vi "subHamamatsu_ApplyDAQwaveform.vi"(5 "Camera info":cluster{"Handle in":u32, "Image file path":path}, 6 "Acquisition params":T1={"Sampling rate (Hz)"=0.0, "dt (sec)"=0.0, "total time (sec)"=0.0, "# samples"=0, "Exposure time (ms)"=1000.0, "# frames"=0} {"Exposure time (ms)" format="%0.5f"; "Sampling rate (Hz)" format="%#.3f"}, 7 "Waveform port selection":T2={"Dev2 DO lines"=["Dev2/port0/line3", "Dev2/port0/line5"], "Dev2 AO lines"=["Dev2/ao3", "Dev2/ao5"], "Patch AO line"="Dev1/ao0", "Dev1 AI lines"=["Dev1/ai0", "Dev1/ai8"], "Dev1 timing DO"="Dev1/port0/line1", "Camera timing DI"="Dev1/port0/line0", "Dev1 trigger source"="/Dev1/PFI0", "Dev2 trigger source"="/Dev2/PFI0"}, 8 "Camera in (no error)":errorcluster, 9 "Dev1 AO waveform":waveform(dbl)(graph)={"t0"=timestamp(0 s since 1904-01-01), "dt"=0.1, "Y"=array[20000 elements]}, 10 "Dev2 AO waveform":waveform(dbl)[](graph)=[{"t0"=timestamp(0 s since 1904-01-01), "dt"=0.1, "Y"=array[20000 elements]}, {"t0"=timestamp(0 s since 1904-01-01), "dt"=0.1, "Y"=array[20000 elements]}], 11 "Dev2 DO waveform":digitalwaveform[](graph)=[{"t0"=timestamp(0 s since 1904-01-01), "dt"=0.1, "Y"={"transitions"=[0, 10000, 19999], "data"=[[1], [0], [0]]}}, {"t0"=timestamp(0 s since 1904-01-01), "dt"=0.1, "Y"={"transitions"=[0, 10000, 19999], "data"=[[0], [1], [1]]}}]) -> (0 "Camera out":errorcluster, 2 "AI Waveform":dbl[][](graph), 3 "Camera timging DI":digitalwaveform(graph))   [LabVIEW 2015]
uses:
  <vilib>/DAQmx/write.llb/DAQmx Write (Analog Wfm 1Chan NSamp).vi
  <vilib>/DAQmx/write.llb/DAQmx Write (Analog 1D Wfm NChan NSamp).vi
  <vilib>/DAQmx/write.llb/DAQmx Write (Digital 1D Wfm NChan NSamp).vi
  <vilib>/DAQmx/write.llb/DAQmx Write (Digital Wfm 1Chan NSamp).vi
  <vilib>/DAQmx/read.llb/DAQmx Read (Analog 2D DBL NChan NSamp).vi
  <vilib>/DAQmx/read.llb/DAQmx Read (Digital Wfm 1Chan NSamp).vi
  <vilib>/DAQmx/create/channels.llb/DAQmx Create Channel (DO-Digital Output).vi
  <vilib>/Waveform/DWDTOps.llb/DWDT Analog to Digital.vi
  <vilib>/DAQmx/create/channels.llb/DAQmx Create Channel (DI-Digital Input).vi
  <vilib>/DAQmx/configure/timing.llb/DAQmx Timing (Sample Clock).vi
  <vilib>/DAQmx/create/channels.llb/DAQmx Create Channel (AO-Voltage-Basic).vi
  <vilib>/DAQmx/miscellaneous.llb/DAQmx Fill In Error Info.vi
  <vilib>/DAQmx/create/channels.llb/DAQmx Create Channel (AI-Voltage-Basic).vi
  <vilib>/DAQmx/configure/trigger.llb/DAQmx Start Trigger (Digital Edge).vi
  <vilib>/Waveform/DWDTOps.llb/DWDT Uncompress Digital.vi
  <vilib>/DAQmx/configure/trigger.llb/DAQmx Start Trigger (None).vi
  <resource>/objmgr/daqmx.rc
panel:
  out "Dev1 SampClk.Rate":dbl format="%#.3f"
  out "Dev2 SampClk.Rate":dbl format="%#.3f"
  out "Dev1 timing DO":digitalwaveform(graph)={"t0"=timestamp(0 s since 1904-01-01), "dt"=0.1, "Y"={"transitions"=[0, 19999], "data"=[[1], [1]]}}
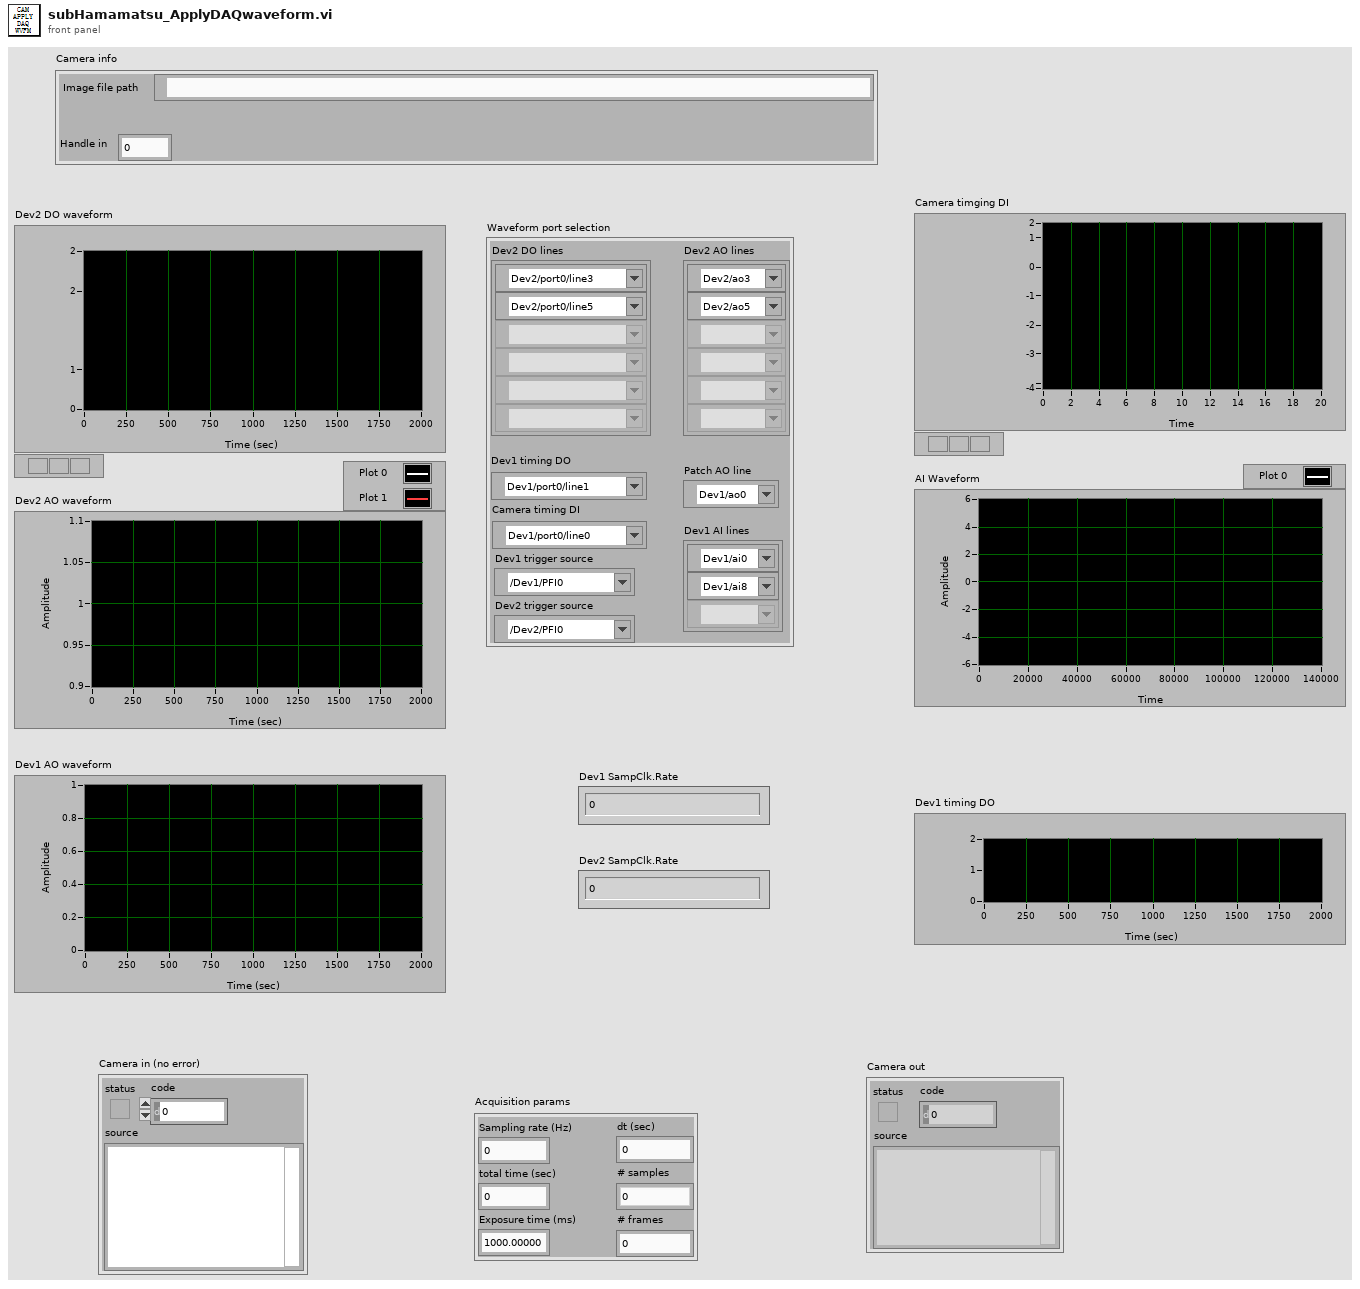
[diagram p1: front panel]
types:
  T1 = cluster{"Sampling rate (Hz)":dbl, "dt (sec)":dbl, "total time (sec)":dbl, "# samples":i32, "Exposure time (ms)":dbl, "# frames":i32}
  T2 = cluster{"Dev2 DO lines":tag[], "Dev2 AO lines":tag[], "Patch AO line":tag, "Dev1 AI lines":tag[], "Dev1 timing DO":tag, "Camera timing DI":tag, "Dev1 trigger source":tag, "Dev2 trigger source":tag}
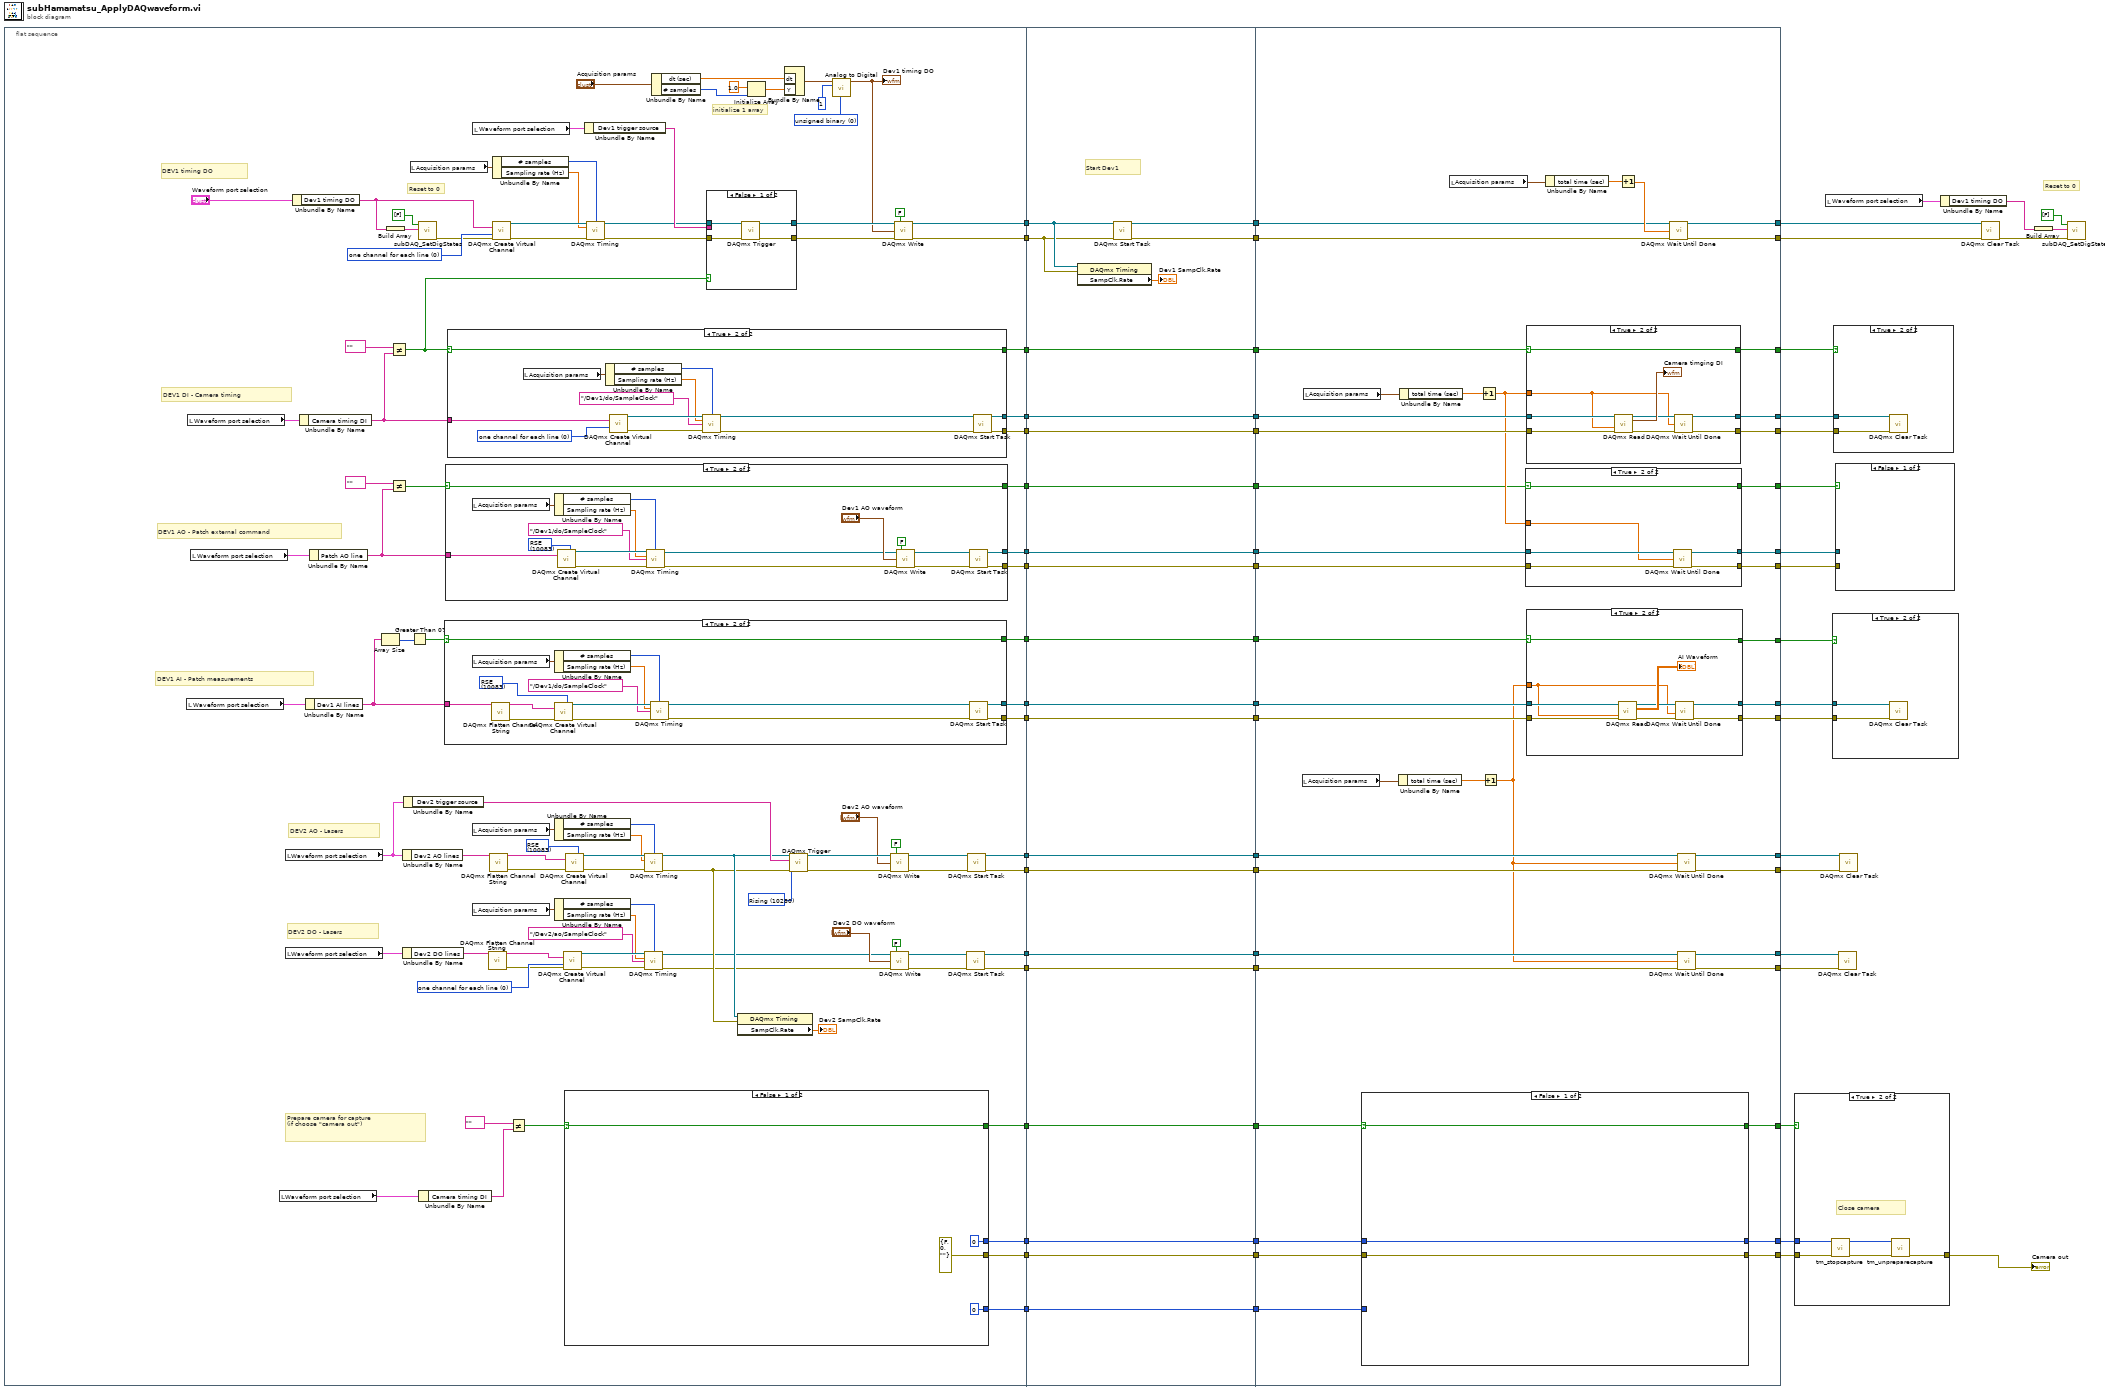
[diagram p0: block diagram]
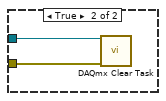
[diagram p5: hidden frame]
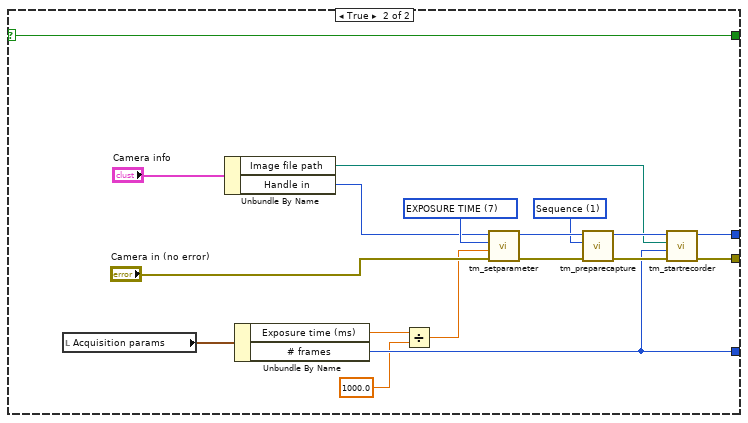
[diagram p6: hidden frame]
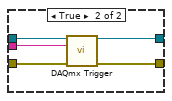
[diagram p7: hidden frame]
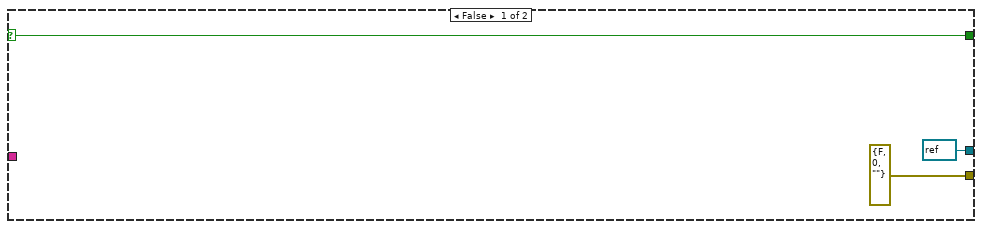
[diagram p8: hidden frame]
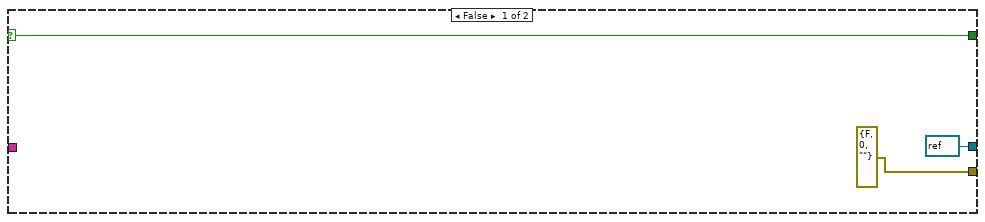
[diagram p9: hidden frame]
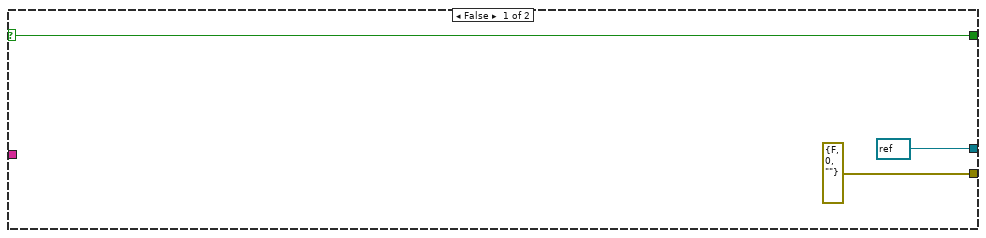
[diagram p10: hidden frame]
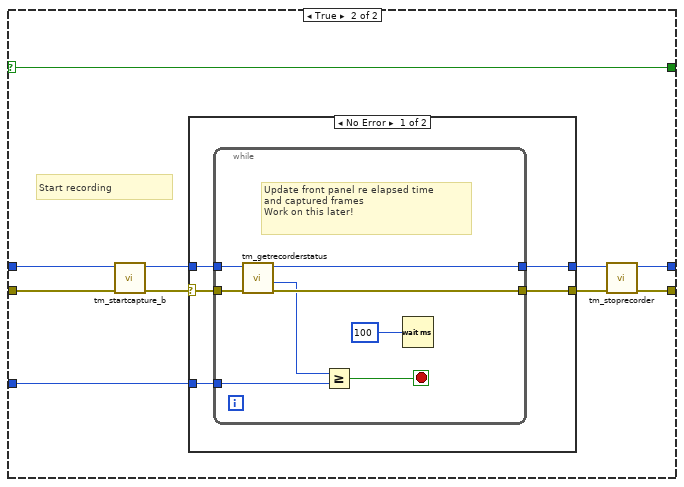
[diagram p11: hidden frame]
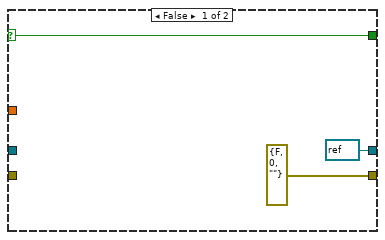
[diagram p13: hidden frame]
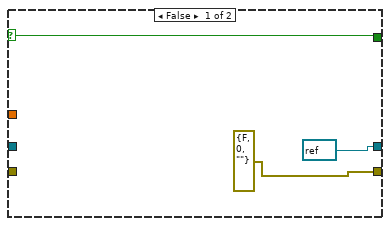
[diagram p14: hidden frame]
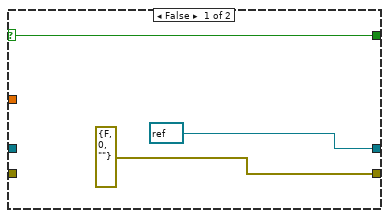
[diagram p15: hidden frame]
diagram:
  # "Reset to 0"
  n1 = flat-sequence {
    tunnel: [w148] -> w39
    tunnel: [w69] -> w37
    tunnel: [w68] -> w35
    tunnel: [w131] -> w34
    tunnel: [w129] -> w32
    tunnel: [w128] -> w30
    tunnel: [w126] -> w28
    tunnel: [w125] -> w26
    tunnel: [w122] -> w24
    tunnel: [w121] -> w22
    tunnel: [w118] -> w20
    tunnel: [w117] -> w18
    tunnel: [w112] -> w16
    tunnel: [w111] -> w14
    tunnel: [w98] -> w12
    tunnel: [w79] -> w10
    tunnel: [w75] -> w8
    tunnel: [w72] -> w6
    tunnel: [w63] -> w2
    tunnel: w39 -> [w269]
    tunnel: [w269] -> w38
    tunnel: w37 -> [w250]
    tunnel: [w252] -> w36
    tunnel: w35 -> [w249]
    tunnel: w34 -> [w268]
    tunnel: [w268] -> w33
    tunnel: w32 -> [w267]
    tunnel: [w267] -> w31
    tunnel: w30 -> [w266]
    tunnel: [w266] -> w29
    tunnel: w28 -> [w265]
    tunnel: [w265] -> w27
    tunnel: w26 -> [w264]
    tunnel: [w264] -> w25
    tunnel: w24 -> [w263]
    tunnel: [w263] -> w23
    tunnel: w22 -> [w262]
    tunnel: [w262] -> w21
    tunnel: w20 -> [w261]
    tunnel: [w261] -> w19
    tunnel: w18 -> [w260]
    tunnel: [w260] -> w17
    tunnel: w16 -> [w259]
    tunnel: [w259] -> w15
    tunnel: w14 -> [w258]
    tunnel: [w258] -> w13
    tunnel: w12 -> [w257]
    tunnel: [w257] -> w11
    tunnel: w10 -> [w256]
    tunnel: [w256] -> w9
    tunnel: w8 -> [w255]
    tunnel: [w255] -> w7
    tunnel: w6 -> [w254]
    tunnel: [w254] -> w5
    tunnel: [w251] -> w4
    tunnel: [w248] -> w3
    tunnel: w2 -> [w248]
    tunnel: w38 -> [w311]
    tunnel: w36 -> [w273]
    tunnel: w33 -> [w310]
    tunnel: w31 -> [w309]
    tunnel: w29 -> [w308]
    tunnel: w27 -> [w306]
    tunnel: w25 -> [w307]
    tunnel: w23 -> [w305]
    tunnel: w21 -> [w304]
    tunnel: w19 -> [w303]
    tunnel: w17 -> [w302]
    tunnel: w15 -> [w315]
    tunnel: w13 -> [w314]
    tunnel: [w313] -> w56
    tunnel: [w312] -> w55
    tunnel: [w301] -> w54
    tunnel: [w300] -> w53
    tunnel: [w299] -> w52
    tunnel: [w298] -> w51
    tunnel: [w297] -> w50
    tunnel: [w296] -> w49
    tunnel: [w295] -> w48
    tunnel: [w294] -> w47
    tunnel: [w293] -> w46
    tunnel: [w292] -> w45
    tunnel: [w291] -> w44
    tunnel: [w290] -> w43
    tunnel: w11 -> [w289]
    tunnel: w9 -> [w279]
    tunnel: [w278] -> w42
    tunnel: w7 -> [w277]
    tunnel: [w276] -> w41
    tunnel: w5 -> [w275]
    tunnel: [w274] -> w40
    tunnel: w4 -> [w272]
    tunnel: w3 -> [w271]
    tunnel: [w270] -> w1
    frame #0 {
      w94 = 10083 items=["Default"=-1, "RSE"=10083, "Differential"=10106, "Pseudodifferential"=12529] ("output terminal configuration")
      w97 = 10280 items=["Rising"=10280, "Falling"=10171] ("edge")
      w110 = u16 0 items=["unsigned binary", "offset binary", "2's complement"] ("data format (offset binary)")
      w140 = 0 items=["one channel for each line", "one channel for all lines"] ("line grouping")
      w162 = 0 items=["one channel for each line", "one channel for all lines"] ("line grouping")
      # "Prepare camera for capture\n(if choose \"camera out\")"
      # "Reset to 0"
      # "DEV2 DO - Lasers"
      # "DEV2 AO - Lasers"
      # "DEV1 AI - Patch measurements"
      # "DEV1 AO - Patch external command"
      # "DEV1 DI - Camera timing"
      # "DEV1 timing DO"
      # "initialize 1 array"
      n2 = local read "Waveform port selection"() -> (w127:T2)
      n3 = local read "Waveform port selection"() -> (w132:T2)
      n4 = local read "Waveform port selection"() -> (w83:T2)
      n5 = local read "Waveform port selection"() -> (w65:T2)
      n6 = local read "Waveform port selection"() -> (w109:T2)
      n7 = local read "Waveform port selection"() -> (w120:T2)
      n8 = Unbundle By Name("Waveform port selection") -> ("Dev1 timing DO"=w115:tag)
      n9 = Unbundle By Name(w132) -> ("Camera timing DI"=w73:tag)
      n10 = Unbundle By Name(w127) -> ("Dev1 AI lines"=w78:tag[])
      n11 = Unbundle By Name(w83) -> ("Patch AO line"=w82:tag)
      n12 = Array Size(array=w78) -> (size(s)=w77:i32)
      n13 = Build Array(w115) -> (w114:tag[])
      n14 = Not Equal?(x=tag "" ("Patch amplifier"), y=w73) -> (x != y?=w70:bool)
      n15 = Not Equal?(x=tag "" ("Patch amplifier"), y=w82) -> (x != y?=w80:bool)
      n16 = Unbundle By Name(w109) -> ("Dev2 AO lines"=w123:tag[])
      n17 = Unbundle By Name(w120) -> ("Dev2 DO lines"=w119:tag[])
      n18 = Unbundle By Name(w109) -> ("Dev2 trigger source"=w108:tag)
      n19 = local read "Acquisition params"() -> (w86:T1)
      n20 = Greater Than 0?(x=w77) -> (x > 0?=w76:bool)
      n21 = call "subDAQ_SetDigStates.vi"("Digital line array"=w114, "Digital States (Value) array"=bool[] [FALSE] ("Digital state array")) -> ("Error out"=w116:errorcluster)  [unwired: 9 in]
      n22 = Unbundle By Name(w65) -> ("Camera timing DI"=w67:tag)
      n23 = case shown="True" w76 {
        selector: w76 -> [w212 w213]
        tunnel: w78 -> [_ w223]
        tunnel: [errorcluster {"status"=FALSE, "code"=0, "source"=""} ("error out") w222] -> w126
        tunnel: [refnum<k21> refnum ("task out") w221] -> w125
        tunnel: [w212 w213] -> w75
        frame False {
        }
        frame True {
          w216 = 10083 items=["Default"=-1, "RSE"=10083, "NRSE"=10078, "Differential"=10106, "Pseudodifferential"=12529] ("input terminal configuration")
          n24 = local read "Acquisition params"() -> (w219:T1)
          n25 = call <vilib>:"DAQmx Flatten Channel String.vi"("names in"=w223) -> ("names out"=w227:string, "error out"=w226:errorcluster)  [unwired: 13 in]
          n26 = Unbundle By Name(w219) -> ("# samples"=w217:i32, "Sampling rate (Hz)"=w218:dbl)
          n27 = call-poly <vilib>:"DAQmx Create Virtual Channel.vi"("input terminal configuration"=w216, "physical channels"=w227, "error in"=w226) -> ("task out"=w224:refnum<k21>, "error out"=w225:errorcluster)  [unwired: 11 in]
          n28 = call-poly <vilib>:"DAQmx Timing.vi"("task/channels in"=w224, "samples per channel"=w217, "rate"=w218, "source"=tag "/Dev1/do/SampleClock", "error in"=w225) -> ("task out"=w215:refnum<k21>, "error out"=w214:errorcluster)  [unwired: 9 in]
          n29 = call <vilib>:"DAQmx Start Task.vi"("task/channels in"=w215, "error in"=w214) -> ("task out"=w221:refnum<k21>, "error out"=w222:errorcluster)  [unwired: 12 in]
        }
      }
      n30 = case shown="True" w80 {
        selector: w80 -> [w230 w231]
        tunnel: [refnum<k21> refnum ("task out") w241] -> w129
        tunnel: [errorcluster {"status"=FALSE, "code"=0, "source"=""} ("error out") w240] -> w128
        tunnel: w82 -> [_ w232]
        tunnel: [w230 w231] -> w79
        frame False {
        }
        frame True {
          w235 = 10083 items=["Default"=-1, "RSE"=10083, "Differential"=10106, "Pseudodifferential"=12529] ("output terminal configuration")
          n31 = local read "Acquisition params"() -> (w236:T1)
          n32 = Unbundle By Name(w236) -> ("# samples"=w238:i32, "Sampling rate (Hz)"=w237:dbl)
          n33 = call-poly <vilib>:"DAQmx Create Virtual Channel.vi"("output terminal configuration"=w235, "physical channels"=w232) -> ("task out"=w244:refnum<k21>, "error out"=w246:errorcluster)  [unwired: 12 in]
          n34 = call-poly <vilib>:"DAQmx Timing.vi"("task/channels in"=w244, "samples per channel"=w238, "rate"=w237, "source"=tag "/Dev1/do/SampleClock", "error in"=w246) -> ("task out"=w234:refnum<k21>, "error out"=w233:errorcluster)  [unwired: 9 in]
          n35 = call-poly <vilib>:"DAQmx Write.vi"("task/channels in"=w234, "auto start"=FALSE, "data"="Dev1 AO waveform", "error in"=w233) -> ("task out"=w245:refnum<k21>, "error out"=w242:errorcluster)  [unwired: 9 in, 1 out]
          n36 = call <vilib>:"DAQmx Start Task.vi"("task/channels in"=w245, "error in"=w242) -> ("task out"=w241:refnum<k21>, "error out"=w240:errorcluster)  [unwired: 12 in]
        }
      }
      n37 = case shown="True" w70 {
        selector: w70 -> [w196 w197]
        tunnel: [refnum<k21> refnum ("task out") w206] -> w148
        tunnel: w73 -> [_ w205]
        tunnel: [errorcluster {"status"=FALSE, "code"=0, "source"=""} ("error out") w204] -> w131
        tunnel: [w196 w197] -> w72
        frame False {
        }
        frame True {
          w209 = 0 items=["one channel for each line", "one channel for all lines"] ("line grouping")
          n38 = local read "Acquisition params"() -> (w202:T1)
          n39 = Unbundle By Name(w202) -> ("# samples"=w201:i32, "Sampling rate (Hz)"=w200:dbl)
          n40 = call-poly <vilib>:"DAQmx Create Virtual Channel.vi"("lines"=w205, "line grouping"=w209) -> ("task out"=w208:refnum<k21>, "error out"=w207:errorcluster)  [unwired: 12 in]
          n41 = call-poly <vilib>:"DAQmx Timing.vi"("task/channels in"=w208, "samples per channel"=w201, "rate"=w200, "source"=tag "/Dev1/do/SampleClock", "error in"=w207) -> ("task out"=w199:refnum<k21>, "error out"=w198:errorcluster)  [unwired: 9 in]
          n42 = call <vilib>:"DAQmx Start Task.vi"("task/channels in"=w199, "error in"=w198) -> ("task out"=w206:refnum<k21>, "error out"=w204:errorcluster)  [unwired: 12 in]
        }
      }
      n43 = local read "Acquisition params"() -> (w104:T1)
      n44 = local read "Acquisition params"() -> (w103:T1)
      n45 = local read "Waveform port selection"() -> (w71:T2)
      n46 = call <vilib>:"DAQmx Flatten Channel String.vi"("names in"=w119) -> ("names out"=w160:string, "error out"=w159:errorcluster)  [unwired: 13 in]
      n47 = call <vilib>:"DAQmx Flatten Channel String.vi"("names in"=w123) -> ("names out"=w144:string, "error out"=w145:errorcluster)  [unwired: 13 in]
      n48 = Unbundle By Name(w86) -> ("# samples"=w85:i32, "Sampling rate (Hz)"=w84:dbl)
      n49 = call-poly <vilib>:"DAQmx Create Virtual Channel.vi"("lines"=w115, "line grouping"=w140, "error in"=w116) -> ("task out"=w141:refnum<k21>, "error out"=w143:errorcluster)  [unwired: 11 in]
      n50 = Not Equal?(x=tag "" ("Patch amplifier"), y=w67) -> (x != y?=w64:bool)
      n51 = Unbundle By Name(w104) -> ("# samples"=w99:i32, "Sampling rate (Hz)"=w100:dbl)
      n52 = Unbundle By Name(w103) -> ("# samples"=w102:i32, "Sampling rate (Hz)"=w101:dbl)
      n53 = call-poly <vilib>:"DAQmx Create Virtual Channel.vi"("lines"=w160, "line grouping"=w162, "error in"=w159) -> ("task out"=w161:refnum<k21>, "error out"=w156:errorcluster)  [unwired: 11 in]
      n54 = case shown="False" w64 {
        selector: w64 -> [w163 w167]
        tunnel: [u32 0 ("Handle out") w177] -> w112
        tunnel: [errorcluster {"status"=FALSE, "code"=0, "source"=""} ("error out") w176] -> w111
        tunnel: [0 ("# frames") w172] -> w98
        tunnel: [w163 w167] -> w63
        frame False {
        }
        frame True {
          w181 = 7 items=["BINNING"=1, "BITS PER CHANNEL"=2, "ACTIVE VIEW INDEX"=3, "CCD MODE"=4, "SENSOR MODE"=5, "READOUT MODE"=6, "EXPOSURE TIME"=7, "CONTRAST GAIN"=8, "CONTRAST OFFSET"=9, "LIGHT MODE"=10, "SENSITIVITY"=11, "WHITE BALANCE"=12, "PHOTON IMAGING MODE"=13, "HIGH DYNAMIC RANGE MODE"=14, "TRIGGER SOURCE"=15, "TRIGGER ACTIVE"=16, "TRIGGER MODE"=17, "TRIGGER POLARITY"=18, "TRIGGER GLOBAL EXPOSURE"=19, "FIRST TRIGGER BEHAVIOR"=20, "TRIGGER TIMES"=21, "OUTPUT TRIGGER POLARITY"=22, "OUTPUT TRIGGER DELAY"=23, "OUTPUT TRIGGER PERIOD"=24, "TEMPERATURE"=25, "TEMPERATURE TARGET"=26, "SENSOR COOLER FAN"=27, "MECHANICAL SHUTTER"=28, "BACK FOCUS POSITION"=29, "FRAMEBUNDLE MODE"=30, "FRAMEBUNDLE NUMBER"=31, "LINEBUNDLE HEIGHT"=32, "TRIGGER CONNECTOR"=33, "IMAGE PIXEL TYPE"=34] ("Parameter")
          w178 = 1 items=["Snap", "Sequence"] ("Capture mode")
          n55 = local read "Acquisition params"() -> (w173:T1)
          n56 = Unbundle By Name("Camera info") -> ("Image file path"=w174:path, "Handle in"=w171:u32)
          n57 = Unbundle By Name(w173) -> ("Exposure time (ms)"=w169:dbl, "# frames"=w172:i32)
          n58 = Divide(x=w169, y=1000.0) -> (x/y=w170:dbl)
          n59 = call "tm_setparameter.vi"("error in (no error)"="Camera in (no error)", "Value in"=w170, "Parameter"=w181, "Handle in"=w171) -> ("error out"=w183:errorcluster, "Handle out"=w182:u32)  [unwired: 6 in]
          n60 = call "tm_preparecapture.vi"("error in (no error)"=w183, "Capture mode"=w178, "Handle in"=w182) -> ("error out"=w179:errorcluster, "Handle out"=w180:u32)  [unwired: 5 in, 2 out]
          n61 = call "tm_startrecorder.vi"("error in (no error)"=w179, "frames"=w172, "File"=w174, "Handle in"=w180) -> ("error out"=w176:errorcluster, "Handle out"=w177:u32)  [unwired: 6 in]
        }
      }
      n62 = call-poly <vilib>:"DAQmx Create Virtual Channel.vi"("output terminal configuration"=w94, "physical channels"=w144, "error in"=w145) -> ("task out"=w155:refnum<k21>, "error out"=w151:errorcluster)  [unwired: 11 in]
      n63 = Unbundle By Name(w71) -> ("Dev1 trigger source"=w106:tag)
      n64 = call-poly <vilib>:"DAQmx Timing.vi"("task/channels in"=w141, "samples per channel"=w85, "rate"=w84, "error in"=w143) -> ("task out"=w90:refnum<k21>, "error out"=w89:errorcluster)  [unwired: 10 in]
      n65 = call-poly <vilib>:"DAQmx Timing.vi"("task/channels in"=w161, "samples per channel"=w102, "rate"=w101, "source"=tag "/Dev2/ao/SampleClock", "error in"=w156) -> ("task out"=w88:refnum<k21>, "error out"=w87:errorcluster)  [unwired: 9 in]
      n66 = call-poly <vilib>:"DAQmx Timing.vi"("task/channels in"=w155, "samples per channel"=w99, "rate"=w100, "error in"=w151) -> ("task out"=w92:refnum<k21>, "error out"=w91:errorcluster)  [unwired: 10 in]
      n67 = Unbundle By Name("Acquisition params") -> ("dt (sec)"=w95:dbl, "# samples"=w96:i32)
      n68 = case shown="False" w70 {
        tunnel: [w186 w193] -> w139
        tunnel: [w187 w192] -> w138
        tunnel: w106 -> [_ w191]
        tunnel: w90 -> [w188 w190]
        tunnel: w89 -> [w185 w189]
        frame False {
          n69 = call-poly <vilib>:"DAQmx Trigger.vi"("task/channels in"=w188, "error in"=w185) -> ("task out"=w187:refnum<k21>, "error out"=w186:errorcluster)  [unwired: 12 in]
        }
        frame True {
          n70 = call-poly <vilib>:"DAQmx Trigger.vi"("task/channels in"=w190, "source"=w191, "error in"=w189) -> ("task out"=w192:refnum<k21>, "error out"=w193:errorcluster)  [unwired: 11 in]
        }
      }
      n71 = property class="DAQmx Timing"(reference=w92, error in=w91) -> ("SampClk.Rate"=→"Dev2 SampClk.Rate":dbl)  [unwired: 2 out]
      n72 = Initialize Array(1.0 ("element"), w96) -> (w136:dbl[])
      n73 = Bundle By Name("dt"=w95, "Y"=w136) -> (w134:waveform(dbl))  [unwired: 1 in]
      n74 = call-poly <vilib>:"DAQmx Trigger.vi"("task/channels in"=w92, "source"=w108, "edge"=w97, "error in"=w91) -> ("task out"=w153:refnum<k21>, "error out"=w152:errorcluster)  [unwired: 10 in]
      n75 = call-poly <vilib>:"Analog to Digital.vi"("data format (offset binary)"=w110, "resolution (16 bit)"=1, "analog waveform"=w134) -> ("digital waveform"=w133:digitalwaveform)  [unwired: 5 in, 3 out]
      "Dev1 timing DO" <- w133
      n76 = call-poly <vilib>:"DAQmx Write.vi"("task/channels in"=w153, "auto start"=FALSE, "data"="Dev2 AO waveform", "error in"=w152) -> ("task out"=w154:refnum<k21>, "error out"=w124:errorcluster)  [unwired: 9 in, 1 out]
      n77 = call-poly <vilib>:"DAQmx Write.vi"("task/channels in"=w88, "auto start"=FALSE, "data"="Dev2 DO waveform", "error in"=w87) -> ("task out"=w158:refnum<k21>, "error out"=w130:errorcluster)  [unwired: 9 in, 1 out]
      n78 = call-poly <vilib>:"DAQmx Write.vi"("task/channels in"=w138, "auto start"=FALSE, "data"=w133, "error in"=w139) -> ("task out"=w69:refnum<k21>, "error out"=w68:errorcluster)  [unwired: 9 in, 1 out]
      n79 = call <vilib>:"DAQmx Start Task.vi"("task/channels in"=w158, "error in"=w130) -> ("task out"=w118:refnum<k21>, "error out"=w117:errorcluster)  [unwired: 12 in]
      n80 = call <vilib>:"DAQmx Start Task.vi"("task/channels in"=w154, "error in"=w124) -> ("task out"=w122:refnum<k21>, "error out"=w121:errorcluster)  [unwired: 12 in]
    }
    frame #1 {
      # "Start Dev1"
      n81 = property class="DAQmx Timing"(reference=w250, error in=w249) -> ("SampClk.Rate"=→"Dev1 SampClk.Rate":dbl)  [unwired: 2 out]
      n82 = call <vilib>:"DAQmx Start Task.vi"("task/channels in"=w250, "error in"=w249) -> ("task out"=w252:refnum<k21>, "error out"=w251:errorcluster)  [unwired: 12 in]
    }
    frame #2 {
      n83 = local read "Acquisition params"() -> (w281:T1)
      n84 = local read "Acquisition params"() -> (w283:T1)
      n85 = case shown="False" w271 {
        selector: w271 -> [w318 w319]
        tunnel: w315 -> [w317 w324]
        tunnel: w314 -> [w316 w323]
        tunnel: [w317 w322] -> w313
        tunnel: [w316 w321] -> w312
        tunnel: w289 -> [_ w320]
        tunnel: [w318 w319] -> w270
        frame False {
        }
        frame True {
          # "Start recording"
          n86 = call "tm_startcapture_b.vi"("error in (no error)"=w323, "Handle in"=w324) -> ("error out"=w325:errorcluster, "Handle out"=w326:u32)  [unwired: 8 in]
          n87 = case shown="No Error" w325 {
            selector: w325 -> [w333 w342]
            tunnel: w326 -> [w332 w343]
            tunnel: [w330 w343] -> w328
            tunnel: [w331 w342] -> w327
            tunnel: w320 -> [w329 _]
            frame No Error {
              n88 = while {
                tunnel: w333 -> [w340]
                tunnel: w332 -> [w339]
                tunnel: [w338] -> w331
                tunnel: [w341] -> w330
                tunnel: w329 -> [w334]
                stop <- w337 stop-if-true
                # "Update front panel re elapsed time\nand captured frames\nWork on this later!"
                n89 = call "tm_getrecorderstatus.vi"("error in (no error)"=w340, "Handle"=w339) -> ("error out"=w338:errorcluster, "Count"=w335:i32, "Handle"=w341:u32)  [unwired: 6 in, 1 out]
                n90 = Greater Or Equal?(x=w335, y=w334) -> (x >= y?=w337:bool)
                n91 = Wait (ms)(milliseconds to wait=u32 100) -> ()  [unwired: 1 out]
              }
            }
            frame Error {
            }
          }
          n92 = call "tm_stoprecorder.vi"("error in (no error)"=w327, "Handle in"=w328) -> ("error out"=w321:errorcluster, "Handle out"=w322:u32)  [unwired: 8 in]
        }
      }
      n93 = Unbundle By Name(w281) -> ("total time (sec)"=w280:dbl)
      n94 = Unbundle By Name(w283) -> ("total time (sec)"=w282:dbl)
      n95 = local read "Acquisition params"() -> (w285:T1)
      n96 = Increment(x=w282) -> (x+1=w287:dbl)
      n97 = Increment(x=w280) -> (x+1=w286:dbl)
      n98 = case shown="True" w279 {
        selector: w279 -> [w370 w372]
        tunnel: w309 -> [_ w376]
        tunnel: w308 -> [_ w375]
        tunnel: [refnum<k21> refnum ("task out") w374] -> w297
        tunnel: [errorcluster {"status"=FALSE, "code"=0, "source"=""} ("error out") w373] -> w296
        tunnel: w287 -> [_ w371]
        tunnel: [w370 w372] -> w278
        frame False {
        }
        frame True {
          n99 = call <vilib>:"DAQmx Wait Until Done.vi"("task/channels in"=w376, "timeout (sec)"=w371, "error in"=w375) -> ("task out"=w374:refnum<k21>, "error out"=w373:errorcluster)  [unwired: 11 in]
        }
      }
      n100 = case shown="True" w275 {
        selector: w275 -> [w346 w347]
        tunnel: w311 -> [_ w352]
        tunnel: w310 -> [_ w351]
        tunnel: [refnum<k21> refnum ("task out") w350] -> w299
        tunnel: [errorcluster {"status"=FALSE, "code"=0, "source"=""} ("error out") w349] -> w298
        tunnel: w287 -> [_ w348]
        tunnel: [w346 w347] -> w274
        frame False {
        }
        frame True {
          n101 = call-poly <vilib>:"DAQmx Read.vi"("task/channels in"=w352, "timeout"=w348, "error in"=w351) -> ("task out"=w353:refnum<k21>, "data"=→"Camera timging DI":digitalwaveform, "error out"=w355:errorcluster)  [unwired: 10 in]
          n102 = call <vilib>:"DAQmx Wait Until Done.vi"("task/channels in"=w353, "timeout (sec)"=w348, "error in"=w355) -> ("task out"=w350:refnum<k21>, "error out"=w349:errorcluster)  [unwired: 11 in]
        }
      }
      n103 = case shown="True" w277 {
        selector: w277 -> [w358 w360]
        tunnel: w307 -> [_ w364]
        tunnel: w306 -> [_ w363]
        tunnel: [refnum<k21> refnum ("task out") w362] -> w295
        tunnel: [errorcluster {"status"=FALSE, "code"=0, "source"=""} ("error out") w361] -> w294
        tunnel: w286 -> [_ w359]
        tunnel: [w358 w360] -> w276
        frame False {
        }
        frame True {
          n104 = call-poly <vilib>:"DAQmx Read.vi"("task/channels in"=w364, "timeout"=w359, "error in"=w363) -> ("task out"=w365:refnum<k21>, "data"=→"AI Waveform":dbl[][], "error out"=w366:errorcluster)  [unwired: 10 in]
          n105 = call <vilib>:"DAQmx Wait Until Done.vi"("task/channels in"=w365, "timeout (sec)"=w359, "error in"=w366) -> ("task out"=w362:refnum<k21>, "error out"=w361:errorcluster)  [unwired: 11 in]
        }
      }
      n106 = Unbundle By Name(w285) -> ("total time (sec)"=w284:dbl)
      n107 = Increment(x=w284) -> (x+1=w288:dbl)
      n108 = call <vilib>:"DAQmx Wait Until Done.vi"("task/channels in"=w273, "timeout (sec)"=w288, "error in"=w272) -> ("task out"=w301:refnum<k21>, "error out"=w300:errorcluster)  [unwired: 11 in]
      n109 = call <vilib>:"DAQmx Wait Until Done.vi"("task/channels in"=w305, "timeout (sec)"=w286, "error in"=w304) -> ("task out"=w293:refnum<k21>, "error out"=w292:errorcluster)  [unwired: 11 in]
      n110 = call <vilib>:"DAQmx Wait Until Done.vi"("task/channels in"=w303, "timeout (sec)"=w286, "error in"=w302) -> ("task out"=w291:refnum<k21>, "error out"=w290:errorcluster)  [unwired: 11 in]
    }
  }
  n111 = case shown="True" w1 {
    tunnel: [w377 w380] -> w57
    tunnel: w56 -> [_ w379]
    tunnel: w55 -> [w377 w378]
    frame False {
    }
    frame True {
      # "Close camera"
      n112 = call "tm_stopcapture.vi"("error in (no error)"=w378, "Handle in"=w379) -> ("error out"=w382:errorcluster, "Handle out"=w381:u32)  [unwired: 8 in]
      n113 = call "tm_unpreparecapture.vi"("error in (no error)"=w382, "Handle in"=w381) -> ("error out"=w380:errorcluster)  [unwired: 8 in, 1 out]
    }
  }
  "Camera out" <- w57
  n114 = local read "Waveform port selection"() -> (w60:T2)
  n115 = case shown="True" w41 {
    tunnel: w48 -> [_ w384]
    tunnel: w47 -> [_ w383]
    frame False {
    }
    frame True {
      n116 = call <vilib>:"DAQmx Clear Task.vi"("task in"=w384, "error in"=w383) -> ()  [unwired: 13 in, 1 out]
    }
  }
  n117 = case shown="True" w40 {
    tunnel: w52 -> [_ w386]
    tunnel: w51 -> [_ w385]
    frame False {
    }
    frame True {
      n118 = call <vilib>:"DAQmx Clear Task.vi"("task in"=w386, "error in"=w385) -> ()  [unwired: 13 in, 1 out]
    }
  }
  n119 = case shown="False" w42 {
    tunnel: w50 -> [_ w388]
    tunnel: w49 -> [_ w387]
    frame False {
    }
    frame True {
      n120 = call <vilib>:"DAQmx Clear Task.vi"("task in"=w388, "error in"=w387) -> ()  [unwired: 13 in, 1 out]
    }
  }
  n121 = call <vilib>:"DAQmx Clear Task.vi"("task in"=w44, "error in"=w43) -> ()  [unwired: 13 in, 1 out]
  n122 = call <vilib>:"DAQmx Clear Task.vi"("task in"=w46, "error in"=w45) -> ()  [unwired: 13 in, 1 out]
  n123 = Unbundle By Name(w60) -> ("Dev1 timing DO"=w58:tag)
  n124 = call <vilib>:"DAQmx Clear Task.vi"("task in"=w54, "error in"=w53) -> ("error out"=w59:errorcluster)  [unwired: 13 in]
  n125 = Build Array(w58) -> (w61:tag[])
  n126 = call "subDAQ_SetDigStates.vi"("Error in (no error)"=w59, "Digital line array"=w61, "Digital States (Value) array"=bool[] [FALSE] ("Digital state array")) -> ()  [unwired: 8 in, 1 out]
